vi "printDocument.vi"(8 "error in (no error)":errorcluster, 10 "printer name (default)":string, 11 "MS-Excel in":refnum<class "MS-Excel.lvclass">) -> (0 "error out":errorcluster, 3 "MS-Excel out":refnum<class "MS-Excel.lvclass">)   [LabVIEW 2017, in "LabVIEW NPOI.lvlib" / "MS-Excel.lvclass"]
uses:
  MS-Excel.lvclass
  <vilib>/registry/registry.llb/Registry RtKey.ctl
  <vilib>/registry/registry.llb/Read Registry Value Simple STR.vi
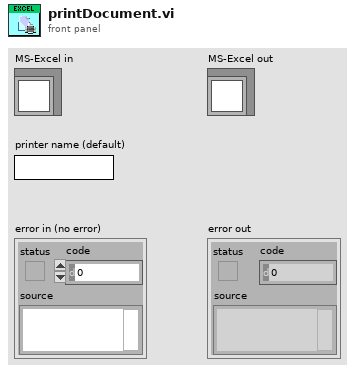
[diagram p1: front panel]
types:
  T1 = typedef "Registry RtKey.ctl" = enum32{"HKEY_CLASSES_ROOT", "HKEY_CURRENT_USER", "HKEY_LOCAL_MACHINE", "HKEY_USERS", "HKEY_PERFORMANCE_DATA", "HKEY_CURRENT_CONFIG", "HKEY_DYN_DATA"}
  T2 = enum32{"KEY_QUERY_VALUE", "KEY_SET_VALUE", "KEY_CREATE_SUB_KEY", "KEY_ENUMERATE_SUB_KEYS", "KEY_NOTIFY", "KEY_CREATE_LINK", "KEY_READ", "KEY_WRITE", "KEY_ALL_ACCESS", "KEY_READ | KEY_WRITE"}
  T3 = typedef "Registry refnum.ctl" = refnum<k1>
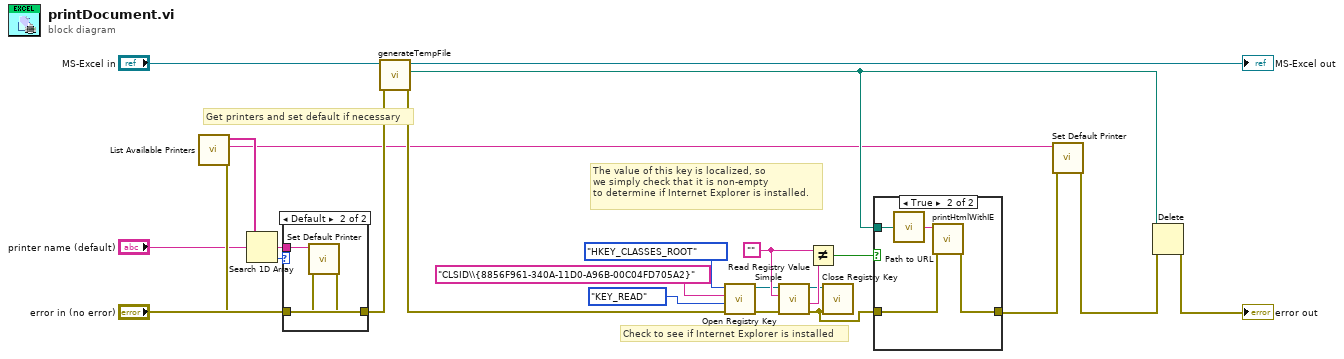
[diagram p0: block diagram]
diagram:
  w21 = ""
  # "Get printers and set default if necessary"
  # "The value of this key is localized, so\nwe simply check that it is non-empty\nto determine if Internet Explorer is installed."
  # "Check to see if Internet Explorer is installed"
  n1 = call "List Available Printers.vi"() -> ("error out"=w6:errorcluster, "Default Printer"=w3:string, "Available Printers"=w7:string[])  [unwired: 9 in]
  n2 = Search 1D Array(1D array=w7, element="printer name (default)") -> (index of element=w5:i32)  [unwired: 1 in]
  n3 = case shown="Default" w5 {
    tunnel: "printer name (default)" -> [_ w25]
    tunnel: w6 -> [w24 w27]
    tunnel: [w24 w26] -> _
    frame -1 {
    }
    frame Default {
      n4 = call "Set Default Printer.vi"("error in (no error)"=w27, "Printer Name"=w25) -> ("error out"=w26:errorcluster)  [unwired: 9 in]
    }
  }
  n5 = call-dynamic "generateTempFile.vi"("error in (no error)"="error in (no error)", "MS-Excel in"="MS-Excel in") -> ("error out"=w8:errorcluster, "Temporary File Path"=w13:path, "MS-Excel out"=→"MS-Excel out":refnum<class "MS-Excel.lvclass">)  [unwired: 7 in]
  n6 = call <vilib>:"Open Registry Key.vi"("error in (no error)"=w8, "security access mask (KEY_READ | KEY_WRITE)"=T2."KEY_READ", "subkey"="CLSID\\{8856F961-340A-11D0-A96B-00C04FD705A2}", "root key (HKEY_LOCAL_MACHINE)"=Registry_RtKey."HKEY_CLASSES_ROOT") -> ("error out"=w18:errorcluster, "refnum out"=w20:T3)  [unwired: 6 out]
  n7 = call-poly <vilib>:"Read Registry Value Simple.vi"("error in (no error)"=w18, "value"=w21, "refnum"=w20) -> ("error out"=w12:errorcluster, "String/Binary data"=w15:string, "refnum out"=w14:T3)  [unwired: 1 in, 3 out]
  n8 = Not Equal?(x=w21, y=w15) -> (x != y?=w11:bool)
  n9 = call <vilib>:"Close Registry Key.vi"("error in (no error)"=w12, "refnum"=w14) -> ()  [unwired: 6 out]
  n10 = case shown="True" w11 {
    tunnel: [w28 w32] -> w2
    tunnel: w13 -> [_ w31]
    tunnel: w12 -> [w28 w29]
    frame False {
    }
    frame True {
      n11 = call <vilib>:"Path to URL.vi"("path"=w31) -> ("url"=w30:string)
      n12 = call "printHtmlWithIE.vi"("error in (no error)"=w29, "path to HTML"=w30) -> ("error out"=w32:errorcluster)  [unwired: 9 in]
    }
  }
  n13 = call "Set Default Printer.vi"("error in (no error)"=w2, "Printer Name"=w3) -> ("error out"=w1:errorcluster)  [unwired: 9 in]
  n14 = Delete(path (use dialog)=w13, error in=w1) -> (error out=→"error out":errorcluster)  [unwired: 3 in, 2 out]
